vi "cluster_strings_to_strict_types.vi"(8 "error in (no error)":errorcluster, 9 "Controls[] (strings)":refnum<vi>[](array[refnum]), 10 "Controls[]":refnum<vi>[](array[refnum])) -> (0 "error out":errorcluster)   [LabVIEW 2018]
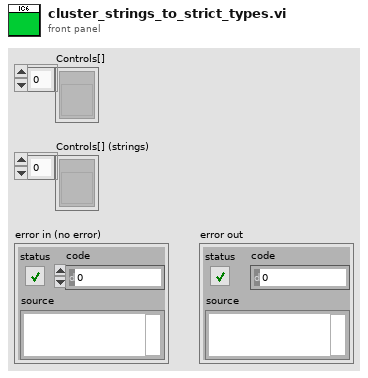
[diagram p1: front panel]
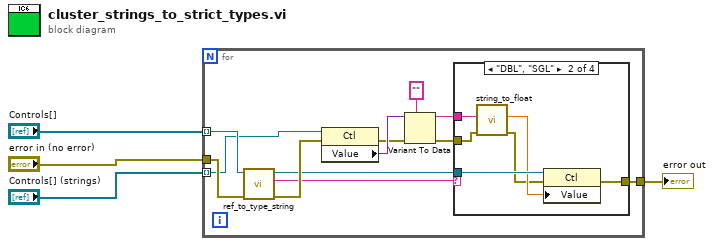
[diagram p0: block diagram]
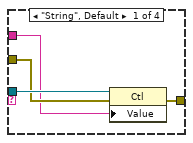
[diagram p2: hidden frame]
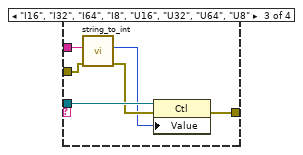
[diagram p3: hidden frame]
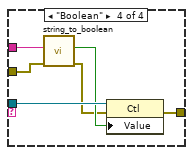
[diagram p4: hidden frame]
diagram:
  n1 = for {
    tunnel: "Controls[]" -> [w6] mode=indexing
    tunnel: "Controls[] (strings)" -> [w5] mode=indexing
    tunnel: "error in (no error)" -> [w10]
    tunnel: [w16] -> w4
    n2 = call "ref_to_type_string.vi"("error in (no error)"=w10, "Control ref in"=w6) -> ("error out"=w9:errorcluster, "Type String"=w7:string, "Control ref out"=w8:refnum<vi>)  [unwired: 7 in]
    n3 = property class="Ctl"(reference=w5, error in=w9) -> (error out=w13:errorcluster, "Value"=w14:variant)  [unwired: 1 out]
    n4 = Variant To Data(error in=w13, type="", Variant=w14) -> (data=w12:string, error out=w11:errorcluster)
    n5 = case shown="\"DBL\", \"SGL\"" w7 {
      tunnel: w8 -> [w20 w26 w32 w38]
      tunnel: [w19 w25 w31 w37] -> w16
      tunnel: w12 -> [w17 w24 w30 w33]
      tunnel: w11 -> [w18 w22 w29 w36]
      frame "String", Default {
        n6 = property class="Ctl"(reference=w20, error in=w18, "Value"=w17) -> (error out=w19:errorcluster)  [unwired: 1 out]
      }
      frame "DBL", "SGL" {
        n7 = call "string_to_float.vi"("error in (no error)"=w22, "Float (string)"=w24) -> ("error out"=w21:errorcluster, "Float (sgl)"=w23:sgl)  [unwired: 8 in]
        n8 = property class="Ctl"(reference=w26, error in=w21, "Value"=w23) -> (error out=w25:errorcluster)  [unwired: 1 out]
      }
      frame "I16", "I32", "I64", "I8", "U16", "U32", "U64", "U8" {
        n9 = call "string_to_int.vi"("error in (no error)"=w29, "Int (string)"=w30) -> ("error out"=w28:errorcluster, "Int"=w27:i32)  [unwired: 8 in]
        n10 = property class="Ctl"(reference=w32, error in=w28, "Value"=w27) -> (error out=w31:errorcluster)  [unwired: 1 out]
      }
      frame "Boolean" {
        n11 = call "string_to_boolean.vi"("error in (no error)"=w36, "Int (string)"=w33) -> ("error out"=w34:errorcluster, "Boolean"=w35:bool)  [unwired: 8 in]
        n12 = property class="Ctl"(reference=w38, error in=w34, "Value"=w35) -> (error out=w37:errorcluster)  [unwired: 1 out]
      }
    }
  }
  "error out" <- w4
